vi "Step_Main.vi"(8 "error in (no error)":errorcluster, 11 "WindmillDevice in":refnum<class "WindmillDevice.lvclass">) -> (0 "error out":errorcluster, 3 "WindmillDevice out":refnum<class "WindmillDevice.lvclass">)   [LabVIEW 2020, in "WindmillDevice.lvclass"]
uses:
  WindmillDevice.lvclass
  WindmillDevice.lvclass/WindmillDevice.ctl
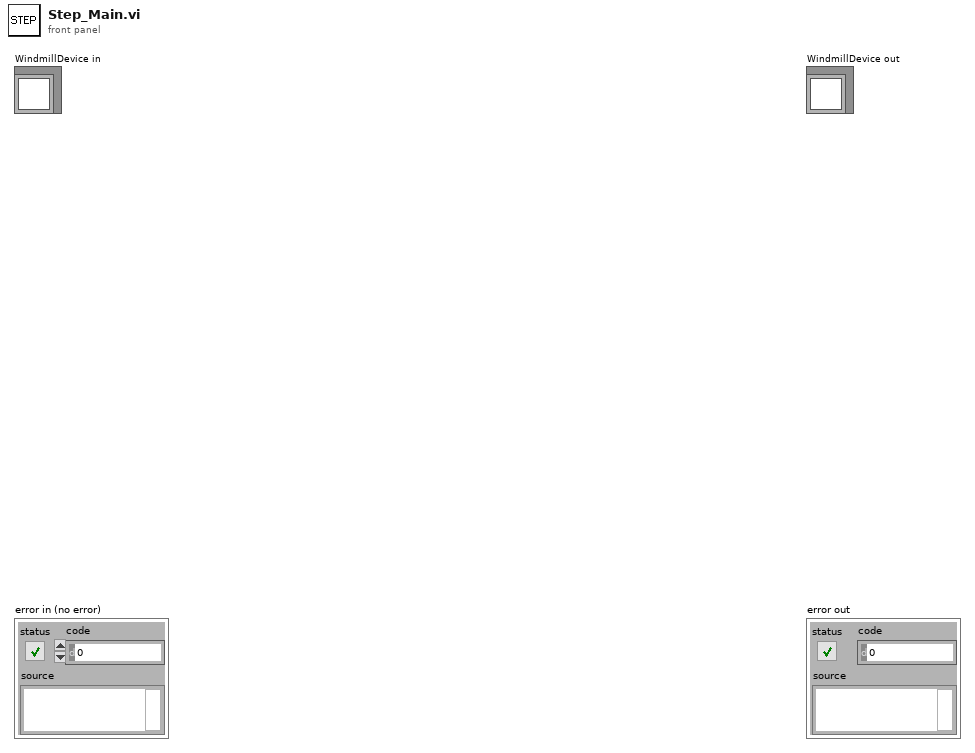
[diagram p1: front panel]
types:
  T1 = typedef "WindmillDevice.lvclass/settingsArcus_TypDef.ctl" = cluster{"device_name":string, "pitch":T2, "position":T2, "lowspeed":T2, "highspeed":T2, "motor_status":enum16{"off", "on"}, "InitDelay":T2, "stepsequence":dbl[], "step":enum16{"off", "on"}, "AutoStep":enum16{"off", "on"}}
  T2 = typedef "BaseDriver.lvclass/numericVariable_TypeDef.ctl" = cluster{"Value":dbl, "Min":dbl, "Max":dbl, "StepSize":dbl, "Tolerance":dbl, "ValueActual":dbl}
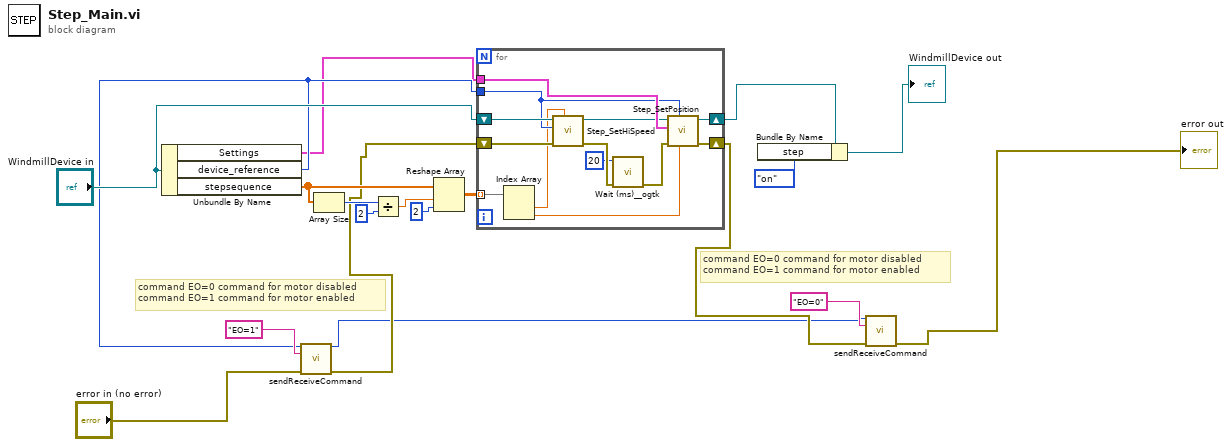
[diagram p0: block diagram]
diagram:
  # "command EO=0 command for motor disabled\ncommand EO=1 command for motor enabled"
  # "command EO=0 command for motor disabled\ncommand EO=1 command for motor enabled"
  n1 = Unbundle By Name("WindmillDevice in") -> ("Settings"=w4:T1, "device_reference"=w5:i32, "stepsequence"=w17:dbl[])
  n2 = call "sendReceiveCommand.vi"("reference (in)"=w5, "write_string"="EO=1", "error in (no error)"="error in (no error)") -> ("reference (out)"=w6:i32, "error out"=w9:errorcluster)  [unwired: 10 in, 1 out]
  n3 = Array Size(array=w17) -> (size(s)=w15:i32)
  n4 = Divide(x=w15, y=2) -> (x/y=w18:dbl)
  n5 = Reshape Array(w17, w18, 2 ("dimension size")) -> (w19:dbl[][])
  n6 = for {
    tunnel: w4 -> [w32]
    tunnel: w5 -> [w26]
    shift-right: [w30] -> w8
    shift-left: w9 -> [w31]
    shift-right: [w27] -> w3
    shift-left: "WindmillDevice in" -> [w29]
    tunnel: w19 -> [w25] mode=indexing
    n7 = Index Array(array=w25) -> (element #1=w24:dbl, element #2=w23:dbl)  [unwired: 2 in]
    n8 = call "Step_SetHiSpeed.vi"("HiSpeed"=w24, "error in (no error)"=w31, "device_reference"=w26, "WindmillDevice in"=w29) -> ("error out"=w22:errorcluster, "WindmillDevice out"=w28:refnum<class "WindmillDevice.lvclass">)  [unwired: 6 in]
    n9 = call "Wait (ms)__ogtk.vi"("error in (no error)"=w22, "milliseconds to wait"=u32 20) -> ("error out"=w21:errorcluster)  [unwired: 8 in, 1 out]
    n10 = call "Step_SetPosition.vi"("Position"=w23, "device_reference"=w26, "error in (no error)"=w21, "Settings"=w32, "WindmillDevice in"=w28) -> ("error out"=w30:errorcluster, "WindmillDevice out"=w27:refnum<class "WindmillDevice.lvclass">)  [unwired: 5 in]
  }
  n11 = Bundle By Name(cluster=w3, "step"=enum16{"off", "on"}."on" ("Settings.step")) -> (→"WindmillDevice out":refnum<class "WindmillDevice.lvclass">)
  n12 = call "sendReceiveCommand.vi"("reference (in)"=w6, "write_string"="EO=0", "error in (no error)"=w8) -> ("error out"=→"error out":errorcluster)  [unwired: 10 in, 2 out]
